vi "readTuplaEnDBProducto.vi"(8 "error in":errorcluster, 11 "claseProducto in":refnum<class "claseProducto.lvclass">) -> (0 "error out":errorcluster, 3 "claseProducto out":refnum<class "claseProducto.lvclass">)   [LabVIEW 2014, in "claseProducto.lvclass"]
uses:
  claseProducto.lvclass
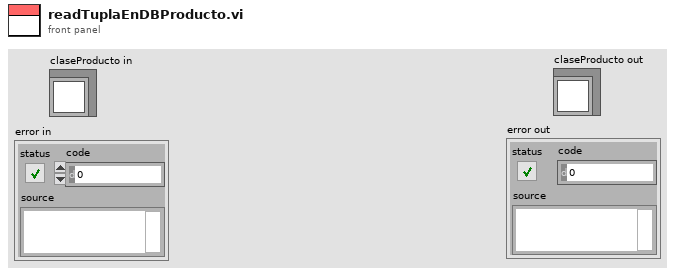
[diagram p1: front panel]
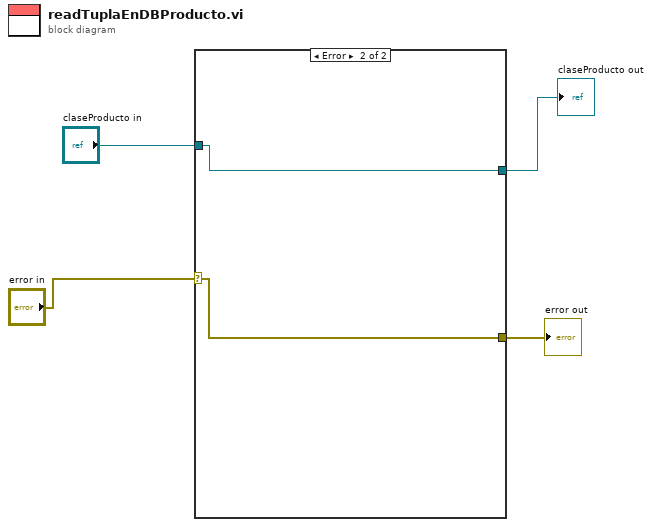
[diagram p0: block diagram]
diagram:
  n1 = case shown="Error" "error in" {
    selector: "error in" -> [w6 w8]
    tunnel: [w6 w8] -> w3
    tunnel: [w5 w7] -> w2
    tunnel: "claseProducto in" -> [w5 w7]
    frame No Error {
    }
    frame Error {
    }
  }
  "claseProducto out" <- w2
  "error out" <- w3
